vi "stopImaging.vi"(8 "error in (no error)":errorcluster, 9 "command_stopImageCapture":T1, 10 "model in":refnum<class "IModel.lvclass">, 11 "CapturingSpectImageState in":refnum<class "CaptureSpectImageState.lvclass">) -> (0 "error out":errorcluster, 2 "model out":refnum<class "IModel.lvclass">, 3 "CapturingSpectImageState out":refnum<class "CaptureSpectImageState.lvclass">)   [LabVIEW 2016, in "States.lvlib" / "CaptureSpectImageState.lvclass"]
uses:
  CaptureSpectImageState.lvclass
  IModel/IModel.lvclass
  ts_sallv_sedspectrometer/DataTypes/command_stopImageCapture.ctl
  Typedefs/CommandValue.ctl
  ts_sallv_sedspectrometer/DataTypes/logevent_DetailedState.ctl
  Typedefs/SEDSpectrometerTypedefs.lvlib
  ts_sallv_sedspectrometer/SALLV_sedSpectrometer.lvlib
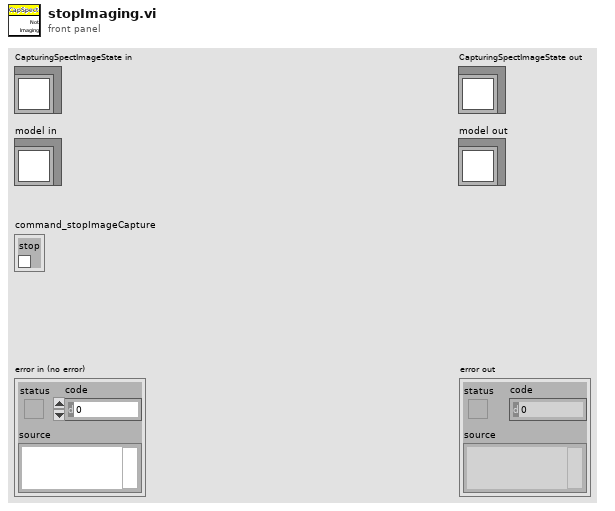
[diagram p1: front panel]
types:
  T1 = typedef "SALLV_sedSpectrometer.lvlib/command_stopImageCapture.ctl" = cluster{"stop":bool}
  T2 = typedef "SALLV_sedSpectrometer.lvlib/logevent_DetailedState.ctl" = cluster{"detailedState":enum32{"", "DisabledState", "EnabledState", "FaultState", "OfflineState", "StandbyState", "CaptureSpectImage", "NotImaging"}, "priority":i32}
  T3 = typedef "SEDSpectrometerTypedefs.lvlib/CommandValue.ctl" = enum16{"disable", "enable", "exit", "GoToStandby", "OnHeartbeat", "OnIncomingMessagingError", "OnInterrupt", "start", "captureSpectImage", "setSpectTempSetpoint", "stopImageCapture"}
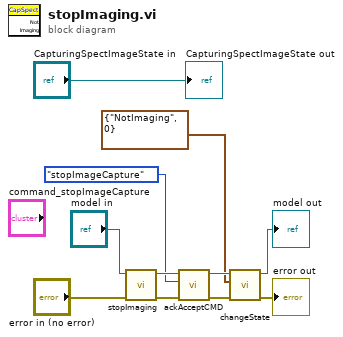
[diagram p0: block diagram]
diagram:
  n1 = call-dynamic "stopImaging.vi"("error in (no error)"="error in (no error)", "IModel in"="model in") -> ("error out"=w3:errorcluster, "IModel out"=w4:refnum<class "IModel.lvclass">)  [unwired: 8 in]
  n2 = call-dynamic "ackAcceptCMD.vi"("error in (no error)"=w3, "CommandValue"=CommandValue."stopImageCapture", "IModel in"=w4) -> ("error out"=w6:errorcluster, "IModel out"=w5:refnum<class "IModel.lvclass">)  [unwired: 7 in]
  n3 = call-dynamic "changeState.vi"("error in (no error)"=w6, "DetailedState"=T2 {"detailedState"=enum."NotImaging", "priority"=0} ("detailedState"), "IModel in"=w5) -> ("error out"=→"error out":errorcluster, "IModel out"=→"model out":refnum<class "IModel.lvclass">)  [unwired: 7 in]
  "CapturingSpectImageState out" <- "CapturingSpectImageState in"
